vi "Configure Power Analysis (Efficiency).vi"(8 "error in (no error)":errorcluster, 11 "VISA resource name":refnum<visa-resource-name>) -> (0 "error out":errorcluster, 3 "VISA resource name out":refnum<visa-resource-name>)   [LabVIEW 2010, in "Agilent 2000 3000 X-Series.lvlib"]
doc: "Applies the effieciency power analysis.\n\n<B>Note(s):</B>\nEfficiency analysis tests the overall efficiency of the power supply by measuring the output power over the input power.\n\nUse <B>Read Measurement (Efficiency Power Analysis).vi</B> to read the result of this power analysis."
uses:
  <instrlib>/Agilent 2000 3000 X-Series/Agilent 2000 3000 X-Series.lvlib
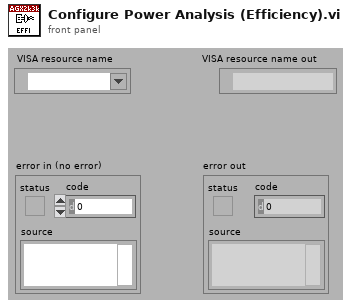
[diagram p1: front panel]
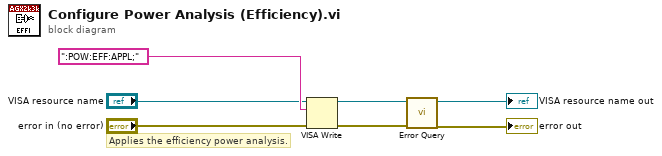
[diagram p0: block diagram]
diagram:
  # "Applies the efficiency power analysis."
  n1 = VISA Write(VISA resource name="VISA resource name", write buffer=":POW:EFF:APPL;", error in (no error)="error in (no error)") -> (VISA resource name out=w4:refnum<visa-resource-name>, error out=w3:errorcluster)  [unwired: 1 out]
  n2 = call <instrlib>:"Error Query.vi"("error in (no error)"=w3, "VISA resource name"=w4) -> ("error out"=→"error out":errorcluster, "VISA resource name out"=→"VISA resource name out":refnum<visa-resource-name>)  [unwired: 8 out]
